vi "Define Panel Actors to Display.vi"(8 "error in (no error)":errorcluster, 10 "panelsEnQrs":refnum<class "Message Enqueuer.lvclass">[](array[class]), 11 "HSplitted in":refnum<class "HSplitted.lvclass">) -> (0 "error out":errorcluster, 3 "HSplitted out":refnum<class "HSplitted.lvclass">)   [LabVIEW 2020, in "HSplitted.lvlib" / "HSplitted.lvclass"]
uses:
  HSplitted.lvclass
  <vilib>/ActorFramework/Message Enqueuer/Message Enqueuer.lvclass
  HSplitted.lvclass/HSplitted.ctl
  <vilib>/MGI/Panel Manager/Panel/Panel/Subpanel/Subpanel.lvclass
  C:/Program Files (x86)/National Instruments/LabVIEW 2020/vi.lib/MGI/Panel Manager/Panel/Panel/Panel.lvclass
  <vilib>/MGI/Panel Manager/Panel Actor/Panel Actor Messages/Change Panel Msg/Change Panel Msg.lvclass
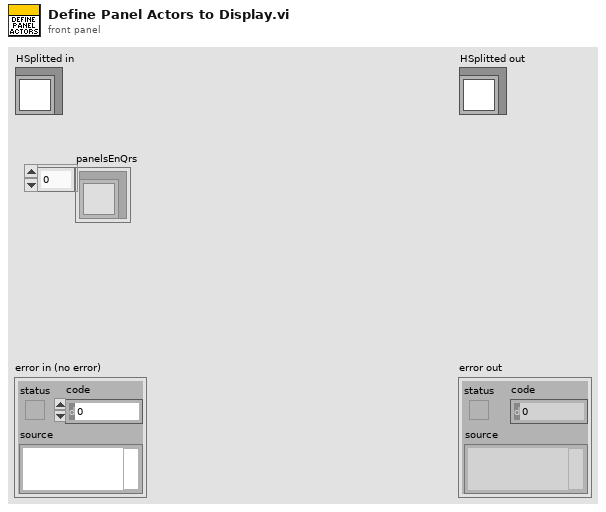
[diagram p1: front panel]
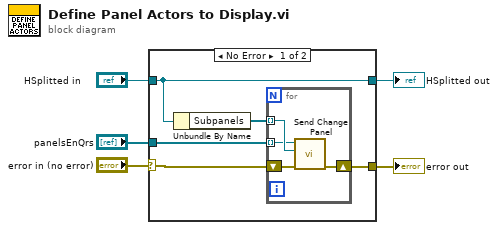
[diagram p0: block diagram]
diagram:
  n1 = case shown="No Error" "error in (no error)" {
    selector: "error in (no error)" -> [w7 w16]
    tunnel: [w6 w16] -> w4
    tunnel: [w10 w15] -> w2
    tunnel: "HSplitted in" -> [w10 w15]
    tunnel: "panelsEnQrs" -> [w8 _]
    frame No Error {
      n2 = Unbundle By Name(w10) -> ("Subpanels"=w9:refnum<class "Subpanel.lvclass">[])
      n3 = for {
        tunnel: w9 -> [w14] mode=indexing
        tunnel: w8 -> [w13] mode=indexing
        shift-right: [w11] -> w6
        shift-left: w7 -> [w12]
        n4 = call <vilib>:"Send Change Panel.vi"("error in (no error)"=w12, "New Panel"=w14, "Message Enqueuer in"=w13) -> ("error out"=w11:errorcluster)  [unwired: 7 in, 1 out]
      }
    }
    frame Error {
    }
  }
  "error out" <- w4
  "HSplitted out" <- w2
